vi "TURCK GUI TestPanel RFID.vi"() -> ()   [LabVIEW 2021]
doc: "Example for reading and writing values for the TBEN-S2-2RFID-4DXP module from Turck"
uses:
  KH TURCK ETHERNETIP TDef Enum RFID Error.ctl
  KH TURCK ETHERNETIP TDefCluster TBEN-S2-2RFID-4DXP Status.ctl
  KH EthernetIPConfig 17.14/KH EthernetIPConfig TDef Config.ctl
  KH EthernetIPConfig 17.14/KH EthernetIPConfig TypeDefs ModuleTyp.ctl
  KH TURCK ETHERNETIP TDefCluster TBEN-S2-2RFID-4DXP Input Values.ctl
  KH TURCK ETHERNETIP TDef Enum RFID User Command.ctl
  KH TURCK TypeDefs FGlob.ctl
  KH EthernetIP 17.19/KH_EthernetIP_Globals.vi
  KH TURCK ETHERNETIP Global.vi
  KH TURCK ETHERNETIP RFID Global.vi
panel:
  out "Status Array":T1[](array[typedef])=[{"Error writing 1"=FALSE, "ReadingFinished 1"=FALSE, "WritingFinished 1"=FALSE, "Error writing 0"=FALSE, "ReadingFinished 0"=FALSE, "WritingFinished 0"=FALSE, "Timeout 1"=FALSE, "State0"="Idle", "State1"="Idle", "Timeout 0"=FALSE, "Successfull Writing 1"=FALSE, "Successfull Writing 0"=FALSE}]
  out "DI":bool[](array[boolean])
  in  "Tab Control":enum32{"Init", " Tag 0", " Tag 1"}(tab)=enum." Tag 1"
  in  "Parameter RFID":T2={"NumberOfBytes0"=312, "SizeFragmentRead1"=128, "SizeFragmentRead0"=128, "SizeFragmentWrite0"=128, "SizeFragmentWrite1"=128, "NumberOfBytes1"=312}
  in  "Config":T3={"Typ"=enum."TBEN-S2-2RFID-4DXP", "Name"="Modul 1", "Nr."=1, "InputOutput"=[enum."Output", enum."Input", enum."Output", enum."Output"]}
  out "UID Tag 0":u8[](array[numeric])
  in  "Write Tag 0":u8[](array[numeric])
  out "Read Tag 0":u8[](array[numeric])
  out "UID Tag 1":u8[](array[numeric])
  in  "Write Tag 1":u8[](array[numeric])
  out "Read Tag 1":u8[](array[numeric])
  in  "Inventory":bool caption="Button"
  in  "Write":bool caption="Button"
  in  "Read":bool caption="Button"
  in  "TagNr":enum16{"Tag 0", "Tag 1"}(ring)
  out "Error1 Modul 1":T5
  out "Error0 Modul 1":T5
  in  "Reset message":bool caption="Button"
  in  "DOS":bool[](array[boolean])=[FALSE, FALSE, FALSE, FALSE]
  out "error out":errorcluster
  in  "Exit":bool
  # "Kirschenhofer Maschinen GmbH\n\n\nRömerstraße 35, 89278 Nersingen-Straß\n\ninfo@kirschenhofer-gmbh.de"
  # "- Before starting the VI your PC has to be in the same subnet as the modules\n- Before starting the VI you have to the change the configuration. You have to change the operation mode into HF extended.\n- You have to set the number of bytes depending of the used tag"
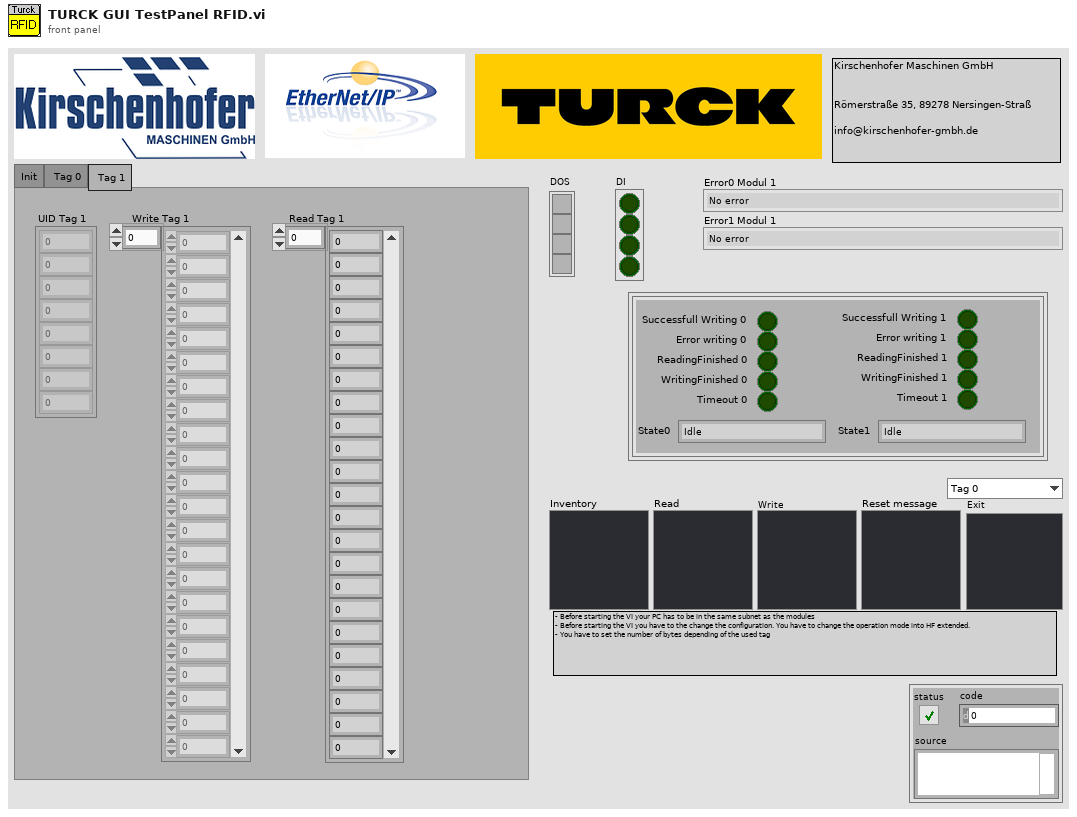
[diagram p1: front panel]
types:
  T1 = typedef "KH TURCK ETHERNETIP TDefCluster TBEN-S2-2RFID-4DXP Status.ctl" = cluster{"Error writing 1":bool, "ReadingFinished 1":bool, "WritingFinished 1":bool, "Error writing 0":bool, "ReadingFinished 0":bool, "WritingFinished 0":bool, "Timeout 1":bool, "State0":string, "State1":string, "Timeout 0":bool, "Successfull Writing 1":bool, "Successfull Writing 0":bool}
  T2 = cluster{"NumberOfBytes0":i32, "SizeFragmentRead1":i32, "SizeFragmentRead0":i32, "SizeFragmentWrite0":i32, "SizeFragmentWrite1":i32, "NumberOfBytes1":i32}
  T3 = typedef "KH EthernetIPConfig TDef Config.ctl" = cluster{"Typ":T4, "Name":string, "Nr.":i32, "InputOutput":enum16{"Input", "Output"}[]}
  T4 = typedef "KH EthernetIPConfig TypeDefs ModuleTyp.ctl" = enum16{"TBEN-S2-4AI", "TBEN-S1-8DXP", "TBEN-S2-2RFID-4DXP", "TBEN-S2-4AO", "TBEN-S2-4IOL"}
  T5 = typedef "KH TURCK ETHERNETIP TDef Enum RFID Error.ctl" = u16
  T6 = typedef "KH TURCK ETHERNETIP TDefCluster TBEN-S2-2RFID-4DXP Input Values.ctl" = cluster{"Station Status Word (Input Data Mapping)":cluster{"Module diagnostics avaliable":bool, "INFO: ARGEE Project Running":bool, "Undervoltage V2":bool, "Undervoltage V1":bool, "Internal Error":bool, "I/O-ASSISTANT Force Mode active":bool}, "RFID control/status 0 (Input Data Mapping)":cluster{"Tag present at r/w head":bool[], "response code":u16, "loop counter":u8, "Length":u16, "Error code":u16, "Tag counter":u16, "Data (Bytes) available":u16, "Read fragment No.":u8, "Write fragment No.":u8, "Tag present at r/w head bit":bool, "HF r/w head switched on":bool, "Continuous mode active":bool, "Antenna detuned at HF read/write head":bool, "Parameter not supported by read/write head":bool, "Error reported by read/write head":bool, "Not connected to read/write head":bool}, "RFID read data 0 (Input Data Mapping)":u8[], "RFID control/status 1 (Input Data Mapping)":cluster{"response code":u16, "Loop counter":u8, "Length":u16, "Error code":u16, "Tag counter":u16, "Data (Bytes) available":u16, "Read fragment No.":u8, "Write fragment No.":u8, "Tag present at r/w head bit":bool, "HF r/w head switched on":bool, "Continuous mode active":bool, "Antenna detuned at HF read/write head":bool, "Parameter not supported by read/write head":bool, "Error reported by read/write head":bool, "Not connected to read/write head":bool, "Tag present at r/w head":bool[]}, "RFID read data 1 (Input Data Mapping)":u8[], "RFID diagnostics (Input Data Mapping)":cluster{"Overcurrent supply VAUX1 (a)":bool, "Parameterization error (a)":bool, "Configuration via DTM active (a)":bool, "Buffer full (a)":bool, "Antenna detuned at HF read/write head (a)":bool[], "Parameter not supported by read/write head (a)":bool[], "Error reported by read/write head (a)":bool[], "Not connected to read/write head (a)":bool[], "Overcurrent supply VAUX1 (b)":bool, "Parameterization error (b)":bool, "Configuration via DTM active (b)":bool, "Buffer full (b)":bool, "Antenna detuned at HF read/write head (b)":bool[], "Parameter not supported by read/write head (b)":bool[], "Error reported by read/write head (b)":bool[], "Not connected to read/write head (b)":bool[]}, "DXP diagnostics (Input Data Mapping)":cluster{"Overcurrent VAUX2 Ch4/5":bool, "Overcurrent VAUX2 Ch6/7":bool, "Channel 4 - Output overcurrent":bool, "Channel 5 - Output overcurrent":bool, "Channel 6 - Output overcurrent":bool, "Channel 7 - Output overcurrent":bool}, "DXP (Input Data Mapping)":cluster{"Channel 4 - Input value":bool, "Channel 5 - Input value":bool, "Channel 6 - Input value":bool, "Channel 7 - Input value":bool}}
  T7 = cluster{"NumberOfBytes0":i32, "SizeFragmentRead1":i32, "SizeFragmentRead0":i32, "SizeFragmentWrite0":i32, "SizeFragmentWrite1":i32, "NumberOfBytes1":i32}[]
  T8 = typedef "KH TURCK ETHERNETIP TDef Enum RFID User Command.ctl" = enum16{"read", "write", "idle", "inventory"}
  T9 = typedef "KH TURCK TypeDefs FGlob.ctl" = enum16{"Put one", "Put all", "Recall one", "Recall all"}
  T10 = typedef "KH TURCK ETHERNETIP TDef Enum RFID Data RFID.ctl" = cluster{"ResponseCode":u16, "LoopCounter":u8, "Length":u16, "WriteFragmentNo":u8, "ReadFragmentNo":u8, "Data":u8[], "TagPresent":bool, "Error":bool, "BusyFinished":bool, "Channel":u16}
  T11 = typedef "KH TURCK ETHERNETIP TDefCluster TURCK RFID.ctl" = cluster{"NumberOfBytes":i32, "State":string, "Counter":i32, "ReadData":u8[], "AnzahlFragmente":i32, "WritingFinished":bool, "ReadingFinished":bool, "UID":u8[], "ActCommand":T12, "SizeFragmentRead":i32, "LengthUID":u16, "WriteDataInclUID":u8[], "Timeout":bool, "SizeFragmentWrite":i32}
  T12 = typedef "KH TURCK ETHERNETIP TDef Enum RFID Act Command.ctl" = enum16{"read", "write", "idle", "Inventory", ""}
  T13 = cluster{"ItemCount":u16, "AdressItem":cluster{"TypeID":u16, "Length":u16, "Data":cluster{"ConnectionIdentifier":u32, "SequenceNumber":u32}}, "DataItem":cluster{"TypeID":u16, "Length":u16, "Data":u8[], "Sequence Count":u16}}
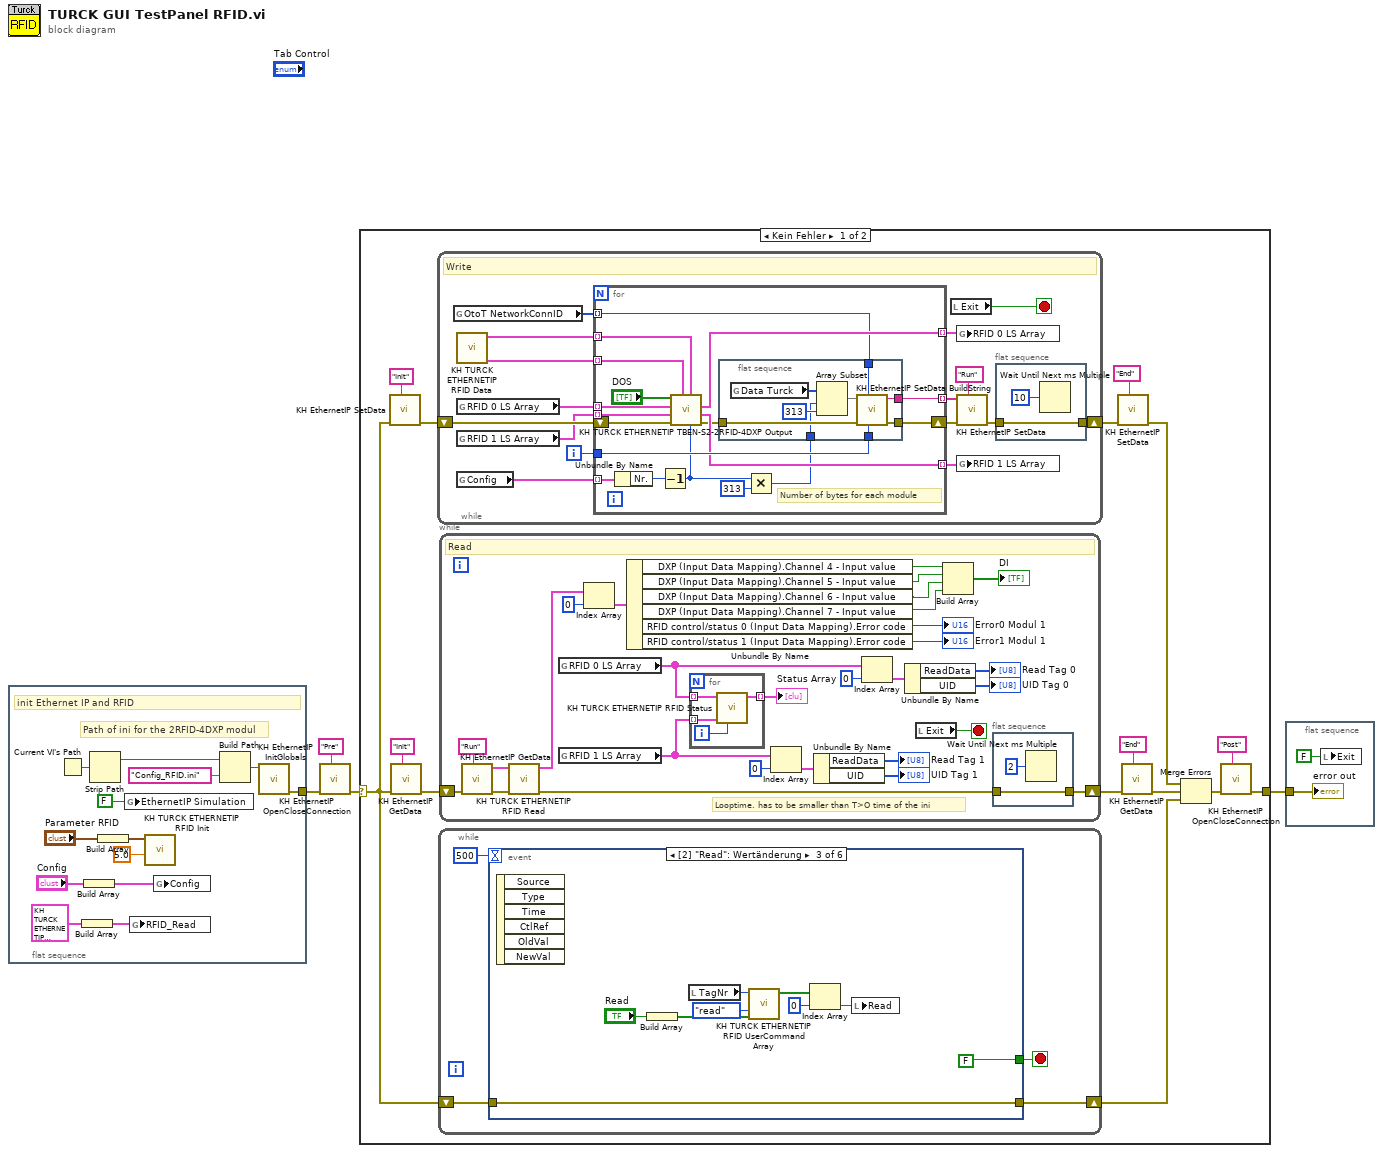
[diagram p0: block diagram]
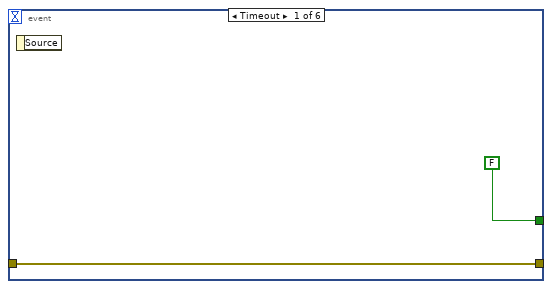
[diagram p2: hidden frame]
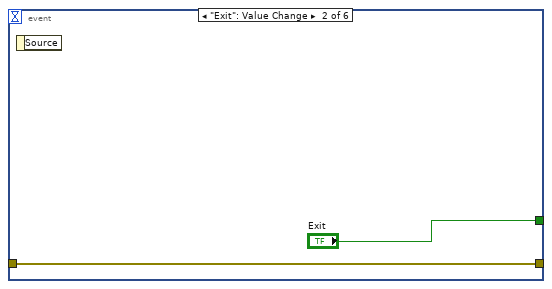
[diagram p3: hidden frame]
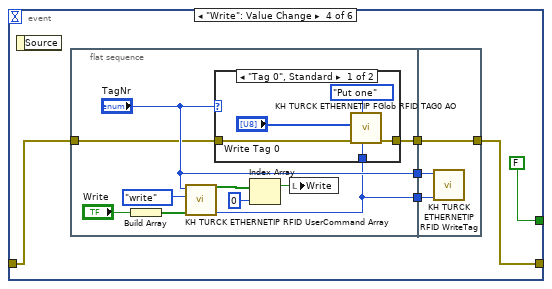
[diagram p4: hidden frame]
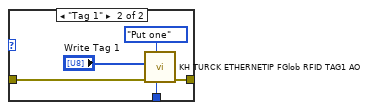
[diagram p5: hidden frame]
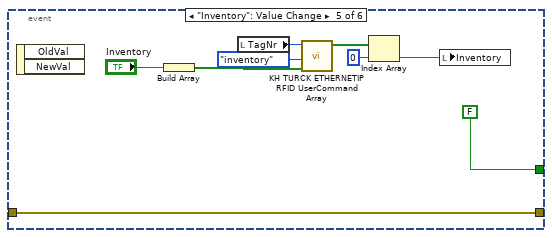
[diagram p6: hidden frame]
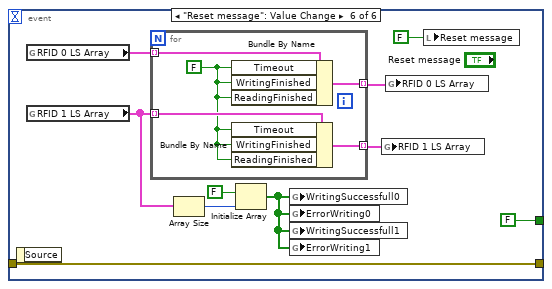
[diagram p7: hidden frame]
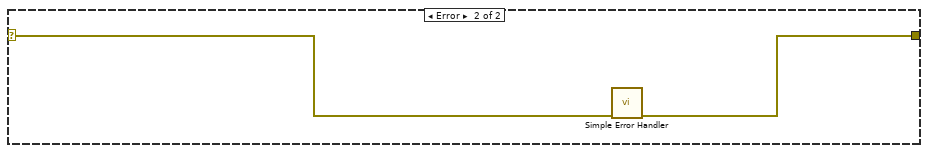
[diagram p8: hidden frame]
diagram:
  n1 = flat-sequence {
    tunnel: [w5] -> w1
    frame #0 {
      # "Path of ini for the 2RFID-4DXP modul"
      # "init Ethernet IP and RFID"
      n2 = Current VI's Path() -> (path=w17:path)
      n3 = Build Array(T6 {"Station Status Word (Input Data Mapping)"={"Module diagnostics avaliable"=FALSE, "INFO: ARGEE Project Running"=FALSE, "Undervoltage V2"=FALSE, "Undervoltage V1"=FALSE, "Internal Error"=FALSE, "I/O-ASSISTANT Force Mode active"=FALSE}, "RFID control/status 0 (Input Data Mapping)"={"Tag present at r/w head"=[], "response code"=0, "loop counter"=0, "Length"=0, "Error code"=0, "Tag counter"=0, "Data (Bytes) available"=0, "Read fragment No."=0, "Write fragment No."=0, "Tag present at r/w head bit"=FALSE, "HF r/w head switched on"=FALSE, "Continuous mode active"=FALSE, "Antenna detuned at HF read/write head"=FALSE, "Parameter not supported by read/write head"=FALSE, "Error reported by read/write head"=FALSE, "Not connected to read/write head"=FALSE}, "RFID read data 0 (Input Data Mapping)"=[], "RFID control/status 1 (Input Data Mapping)"={"response code"=0, "Loop counter"=0, "Length"=0, "Error code"=0, "Tag counter"=0, "Data (Bytes) available"=0, "Read fragment No."=0, "Write fragment No."=0, "Tag present at r/w head bit"=FALSE, "HF r/w head switched on"=FALSE, "Continuous mode active"=FALSE, "Antenna detuned at HF read/write head"=FALSE, "Parameter not supported by read/write head"=FALSE, "Error reported by read/write head"=FALSE, "Not connected to read/write head"=FALSE, "Tag present at r/w head"=[]}, "RFID read data 1 (Input Data Mapping)"=[], "RFID diagnostics (Input Data Mapping)"={"Overcurrent supply VAUX1 (a)"=FALSE, "Parameterization error (a)"=FALSE, "Configuration via DTM active (a)"=FALSE, "Buffer full (a)"=FALSE, "Antenna detuned at HF read/write head (a)"=[], "Parameter not supported by read/write head (a)"=[], "Error reported by read/write head (a)"=[], "Not connected to read/write head (a)"=[], "Overcurrent supply VAUX1 (b)"=FALSE, "Parameterization error (b)"=FALSE, "Configuration via DTM active (b)"=FALSE, "Buffer full (b)"=FALSE, "Antenna detuned at HF read/write head (b)"=[], "Parameter not supported by read/write head (b)"=[], "Error reported by read/write head (b)"=[], "Not connected to read/write head (b)"=[]}, "DXP diagnostics (Input Data Mapping)"={"Overcurrent VAUX2 Ch4/5"=FALSE, "Overcurrent VAUX2 Ch6/7"=FALSE, "Channel 4 - Output overcurrent"=FALSE, "Channel 5 - Output overcurrent"=FALSE, "Channel 6 - Output overcurrent"=FALSE, "Channel 7 - Output overcurrent"=FALSE}, "DXP (Input Data Mapping)"={"Channel 4 - Input value"=FALSE, "Channel 5 - Input value"=FALSE, "Channel 6 - Input value"=FALSE, "Channel 7 - Input value"=FALSE}} ("element")) -> (w7:T6[])
      n4 = Build Array("Config") -> (w8:T3[])
      n5 = Strip Path(path=w17) -> (stripped path=w16:path)  [unwired: 1 out]
      n6 = Build Array("Parameter RFID") -> (w11:T7)
      n7 = global write "KH_EthernetIP_Globals.vi" "EthernetIP Simulation"(FALSE ("EthernetIP Simulation")) -> ()
      n8 = global write "KH TURCK ETHERNETIP Global.vi" "RFID_Read"(w7) -> ()
      n9 = call "KH TURCK ETHERNETIP RFID Init.vi"("Timeout"=5.0, "Parameter RFID Array"=w11) -> ()  [unwired: 9 in, 1 out]
      n10 = global write "KH_EthernetIP_Globals.vi" "Config"(w8) -> ()
      n11 = Build Path(base path=w16, name or relative path="Config_RFID.ini") -> (appended path=w14:path)
      n12 = call "KH EthernetIP InitGlobals.vi"("Config File"=w14) -> ("err out"=w5:errorcluster)  [unwired: 10 in]
    }
  }
  n13 = call "KH EthernetIP OpenCloseConnection.vi"("Function"="Pre", "error in"=w1) -> ("error out"=w3:errorcluster)  [unwired: 9 in]
  n14 = case shown="Kein Fehler" w3 {
    selector: w3 -> [w18 w183]
    tunnel: [w19 w182] -> w2
    frame No Error {
      n15 = call "KH EthernetIP SetData.vi"("Function"="Init", "error in"=w18) -> ("error out"=w22:errorcluster)  [unwired: 7 in, 2 out]
      n16 = call "KH EthernetIP GetData.vi"("Function"="Init", "error in"=w18) -> ("error out"=w32:errorcluster)  [unwired: 8 in, 1 out]
      n17 = while {
        shift-right: [w46] -> w23
        shift-left: w22 -> [w44]
        i -> [w43]
        stop <- w42 stop-if-true
        # "Write"
        n18 = global read "KH_EthernetIP_Globals.vi" "OtoT NetworkConnID"() -> (w33:u32[])
        n19 = call "KH TURCK ETHERNETIP RFID Data.vi"() -> ("RFID 0 Read SM"=w35:T10[], "RFID 1 Read SM"=w36:T10[])  [unwired: 10 in]
        n20 = global read "KH TURCK ETHERNETIP RFID Global.vi" "RFID 0 LS Array"() -> (w38:T11[])
        n21 = global read "KH TURCK ETHERNETIP RFID Global.vi" "RFID 1 LS Array"() -> (w40:T11[])
        n22 = global read "KH_EthernetIP_Globals.vi" "Config"() -> (w34:T3[])
        n23 = for {
          tunnel: [w65] -> w41 mode=indexing
          tunnel: w43 -> [w63]
          shift-right: [w66] -> w45
          shift-left: w44 -> [w64]
          tunnel: w36 -> [w54] mode=indexing
          tunnel: w35 -> [w55] mode=indexing
          tunnel: w38 -> [w60] mode=indexing
          tunnel: w40 -> [w62] mode=indexing
          tunnel: [w61] -> w39 mode=indexing
          tunnel: [w59] -> w37 mode=indexing
          tunnel: w34 -> [w52] mode=indexing
          tunnel: w33 -> [w49] mode=indexing
          # "Number of bytes for each module"
          n24 = Unbundle By Name(w52) -> ("Nr."=w53:i32)
          n25 = Decrement(x=w53) -> (x-1=w50:i32)
          n26 = call "KH TURCK ETHERNETIP TBEN-S2-2RFID-4DXP Output.vi"("Nr Modul"=w50, "Read 1 SM"=w54, "Read 0 SM"=w55, "error in"=w64, "ReadWrite 1 SM In"=w62, "ReadWrite 0 SM In"=w60, "RFID DXP"="DOS") -> ("error out"=w58:errorcluster, "ReadWrite 1 SM Out"=w61:T11, "ReadWrite 0 SM Out"=w59:T11)  [unwired: 1 in, 1 out]
          n27 = flat-sequence {
            tunnel: [w75] -> w66
            tunnel: w49 -> [w74]
            tunnel: [w73] -> w65
            tunnel: w63 -> [w72]
            tunnel: w58 -> [w70]
            tunnel: w57 -> [w69]
            frame #0 {
              n28 = global read "KH TURCK ETHERNETIP Global.vi" "Data Turck"() -> (w67:u8[])
              n29 = Array Subset(array=w67, index=w69, length=313) -> (w68:u8[])
              n30 = call "KH EthernetIP SetData BuildString.vi"("LoopIndex"=w72, "OtoT NetworkConnID"=w74, "error in"=w70, "Output Data"=w68) -> ("error out"=w75:errorcluster, "DataString"=w73:string)  [unwired: 6 in]
            }
          }
          n31 = Multiply(x=w50, y=313) -> (x*y=w57:i32)
        }
        n32 = local read "Exit"() -> (w42:bool)
        n33 = global write "KH TURCK ETHERNETIP RFID Global.vi" "RFID 0 LS Array"(w37) -> ()
        n34 = call "KH EthernetIP SetData.vi"("Function"="Run", "error in"=w45, "Data Strings"=w41) -> ("error out"=w47:errorcluster)  [unwired: 6 in, 2 out]
        n35 = global write "KH TURCK ETHERNETIP RFID Global.vi" "RFID 1 LS Array"(w39) -> ()
        n36 = flat-sequence {
          tunnel: w47 -> [w76]
          tunnel: [w76] -> w46
          frame #0 {
            n37 = Wait Until Next ms Multiple(millisecond multiple=u32 10) -> ()  [unwired: 1 out]
          }
        }
      }
      n38 = while {
        shift-right: [w112] -> w20
        shift-left: w18 -> [w114]
        stop <- w115 stop-if-true
        n39 = event shown="[2] \"Read\": Wertänderung" {
          selector: _ -> [_ _ _ _ _ _]
          dyn-events: _ -> [_ _ _ _ _ _]
          timeout: 500 -> [_ _ _ _ _ _]
          tunnel: [FALSE ("Exit") "Exit" FALSE ("Exit") FALSE ("Exit") FALSE ("Exit") FALSE ("Exit")] -> w115
          tunnel: w114 -> [w116 w118 w127 w133 w165 w175]
          tunnel: [w116 w118 w127 w132 w165 w175] -> w112
          event Timeout {
            n40 = event-data() -> ()  [unwired: 1 in, 1 out]
          }
          event "Exit": Value Change {
            n41 = event-data() -> ()  [unwired: 1 in, 1 out]
          }
          event "Read": Value Change {
            n42 = event-data() -> ()  [unwired: 1 in, 6 out]
            n43 = Build Array("Read") -> (w123:bool[])
            n44 = local read "TagNr"() -> (w126:enum16{"Tag 0", "Tag 1"})
            n45 = call "KH TURCK ETHERNETIP RFID UserCommand Array.vi"("BitArray"=w123, "UserCommand"=KH_TURCK_ETHERNETIP_TDef_Enum_RFID_User_Command."read", "TagNr"=w126) -> ("initialized array"=w122:bool[])  [unwired: 7 in, 1 out]
            n46 = Index Array(array=w122, index=0) -> (element=w120:bool)
            n47 = local write "Read"(w120) -> ()
          }
          event "Write": Value Change {
            n48 = event-data() -> ()  [unwired: 1 in, 1 out]
            n49 = flat-sequence {
              tunnel: w133 -> [w141]
              tunnel: [w142] -> w131
              tunnel: ["TagNr"] -> w130
              tunnel: [w135] -> w129
              tunnel: [w157] -> w132
              tunnel: w131 -> [w157]
              tunnel: w130 -> [w156]
              tunnel: w129 -> [w155]
              frame #0 {
                n50 = Build Array("Write") -> (w139:bool[])
                n51 = call "KH TURCK ETHERNETIP RFID UserCommand Array.vi"("BitArray"=w139, "UserCommand"=KH_TURCK_ETHERNETIP_TDef_Enum_RFID_User_Command."write", "TagNr"="TagNr") -> ("index of element"=w135:i32, "initialized array"=w137:bool[])  [unwired: 7 in]
                n52 = case shown="\"Tag 0\", Standard" "TagNr" {
                  tunnel: [w147 w154] -> w142
                  tunnel: w141 -> [w146 w153]
                  tunnel: w135 -> [w145 w150]
                  frame "Tag 0", Default {
                    n53 = call "KH TURCK ETHERNETIP FGlob RFID TAG0 AO.vi"("Nr Module"=w145, "Function"=KH_TURCK_TypeDefs_FGlob."Put one", "err in"=w146, "RFID one in"="Write Tag 0") -> ("err out"=w147:errorcluster)  [unwired: 5 in, 2 out]
                  }
                  frame "Tag 1" {
                    n54 = call "KH TURCK ETHERNETIP FGlob RFID TAG1 AO.vi"("Nr Module"=w150, "Function"=KH_TURCK_TypeDefs_FGlob."Put one", "err in"=w153, "RFID one in"="Write Tag 1") -> ("err out"=w154:errorcluster)  [unwired: 5 in, 2 out]
                  }
                }
                n55 = Index Array(array=w137, index=0) -> (element=w136:bool)
                n56 = local write "Write"(w136) -> ()
              }
              frame #1 {
                n57 = call "KH TURCK ETHERNETIP RFID WriteTag.vi"("Modul Nr"=w155, "TagNr"=w156) -> ()  [unwired: 10 in]
              }
            }
          }
          event "Inventory": Value Change {
            n58 = event-data() -> ()  [unwired: 1 in, 2 out]
            n59 = Build Array("Inventory") -> (w161:bool[])
            n60 = local read "TagNr"() -> (w164:enum16{"Tag 0", "Tag 1"})
            n61 = call "KH TURCK ETHERNETIP RFID UserCommand Array.vi"("BitArray"=w161, "UserCommand"=KH_TURCK_ETHERNETIP_TDef_Enum_RFID_User_Command."inventory", "TagNr"=w164) -> ("initialized array"=w160:bool[])  [unwired: 7 in, 1 out]
            n62 = Index Array(array=w160, index=0) -> (element=w159:bool)
            n63 = local write "Inventory"(w159) -> ()
          }
          event "Reset message": Value Change {
            n64 = event-data() -> ()  [unwired: 1 in, 1 out]
            n65 = global read "KH TURCK ETHERNETIP RFID Global.vi" "RFID 0 LS Array"() -> (w169:T11[])
            n66 = global read "KH TURCK ETHERNETIP RFID Global.vi" "RFID 1 LS Array"() -> (w168:T11[])
            n67 = for {
              tunnel: [w180] -> w173 mode=indexing
              tunnel: w169 -> [w181] mode=indexing
              tunnel: w168 -> [w179] mode=indexing
              tunnel: [w177] -> w167 mode=indexing
              w178 = FALSE ("TimeoutReading")
              n68 = Bundle By Name(cluster=w181, "Timeout"=w178, "WritingFinished"=w178, "ReadingFinished"=w178) -> (w180:T11)
              n69 = Bundle By Name(cluster=w179, "Timeout"=w178, "WritingFinished"=w178, "ReadingFinished"=w178) -> (w177:T11)
            }
            n70 = Array Size(array=w168) -> (size(s)=w172:i32)
            n71 = Initialize Array(FALSE ("TimeoutReading"), w172) -> (w170:bool[])
            n72 = global write "KH TURCK ETHERNETIP RFID Global.vi" "WritingSuccessfull0"(w170) -> ()
            n73 = global write "KH TURCK ETHERNETIP RFID Global.vi" "ErrorWriting0"(w170) -> ()
            n74 = global write "KH TURCK ETHERNETIP RFID Global.vi" "WritingSuccessfull1"(w170) -> ()
            n75 = global write "KH TURCK ETHERNETIP RFID Global.vi" "ErrorWriting1"(w170) -> ()
            n76 = global write "KH TURCK ETHERNETIP RFID Global.vi" "RFID 1 LS Array"(w167) -> ()
            n77 = global write "KH TURCK ETHERNETIP RFID Global.vi" "RFID 0 LS Array"(w173) -> ()
            n78 = local write "Reset message"(FALSE ("TimeoutWriting")) -> ()
          }
        }
      }
      n79 = while {
        shift-right: [w103] -> w30
        shift-left: w32 -> [w105]
        stop <- w99 stop-if-true
        # "Looptime. has to be smaller than T>O time of the ini"
        # "Read"
        n80 = call "KH EthernetIP GetData.vi"("Function"="Run", "error in"=w105) -> ("error out"=w80:errorcluster, "Response Data"=w81:T13)  [unwired: 8 in]
        n81 = call "KH TURCK ETHERNETIP RFID Read.vi"("error in"=w80, "Response Data"=w81) -> ("error out"=w78:errorcluster, "RFID_Read"=w79:T6[])  [unwired: 8 in]
        n82 = global read "KH TURCK ETHERNETIP RFID Global.vi" "RFID 0 LS Array"() -> (w92:T11[])
        n83 = global read "KH TURCK ETHERNETIP RFID Global.vi" "RFID 1 LS Array"() -> (w87:T11[])
        n84 = Index Array(array=w79, index=0) -> (element=w95:T6)
        n85 = Unbundle By Name(w95) -> ("DXP (Input Data Mapping).Channel 4 - Input value"=w86:bool, "DXP (Input Data Mapping).Channel 5 - Input value"=w85:bool, "DXP (Input Data Mapping).Channel 6 - Input value"=w84:bool, "DXP (Input Data Mapping).Channel 7 - Input value"=w83:bool, "RFID control/status 0 (Input Data Mapping).Error code"=→"Error0 Modul 1":u16, "RFID control/status 1 (Input Data Mapping).Error code"=→"Error1 Modul 1":u16)
        n86 = for {
          tunnel: w92 -> [w109] mode=indexing
          tunnel: w87 -> [w108] mode=indexing
          tunnel: [w107] -> w98 mode=indexing
          i -> [w106]
          n87 = call "KH TURCK ETHERNETIP RFID Status.vi"("Nr.Module"=w106, "RFID 1"=w108, "RFID 0"=w109) -> ("StatusOUT"=w107:T1)  [unwired: 8 in]
        }
        "Status Array" <- w98
        n88 = Index Array(array=w87, index=0) -> (element=w90:T11)
        n89 = Unbundle By Name(w90) -> ("ReadData"=→"Read Tag 1":u8[], "UID"=→"UID Tag 1":u8[])
        n90 = Index Array(array=w92, index=0) -> (element=w96:T11)
        n91 = Unbundle By Name(w96) -> ("ReadData"=→"Read Tag 0":u8[], "UID"=→"UID Tag 0":u8[])
        n92 = local read "Exit"() -> (w99:bool)
        n93 = Build Array(w86, w85, w84, w83) -> (→"DI":bool[])
        n94 = flat-sequence {
          tunnel: w78 -> [w110]
          tunnel: [w110] -> w103
          frame #0 {
            n95 = Wait Until Next ms Multiple(millisecond multiple=u32 2) -> ()  [unwired: 1 out]
          }
        }
      }
      n96 = call "KH EthernetIP SetData.vi"("Function"="End", "error in"=w23) -> ("error out"=w27:errorcluster)  [unwired: 7 in, 2 out]
      n97 = call "KH EthernetIP GetData.vi"("Function"="End", "error in"=w30) -> ("error out"=w25:errorcluster)  [unwired: 8 in, 1 out]
      n98 = Merge Errors(w27, w25, w20) -> (w26:errorcluster)
      n99 = call "KH EthernetIP OpenCloseConnection.vi"("Function"="Post", "error in"=w26) -> ("error out"=w19:errorcluster)  [unwired: 9 in]
    }
    frame Error {
      n100 = call <vilib>:"Simple Error Handler.vi"("error in (no error)"=w183) -> ("error out"=w182:errorcluster)  [unwired: 4 in, 4 out]
    }
  }
  n101 = flat-sequence {
    tunnel: w2 -> [w184]
    frame #0 {
      n102 = local write "Exit"(FALSE ("Exit")) -> ()
      "error out" <- w184
    }
  }
